vi "Calculate_aomVolts.vi"(8 "error in (no error)":errorcluster, 10 "Power":dbl[](array[numeric])=[0.0, 0.0, 0.0, 0.0] min=0.0 max=1.0, 11 "Fit Parameters":dbl[](array[numeric])=[0.16846, 70.4259, 1.31931]) -> (0 "error out":errorcluster, 2 "AOM Voltage":dbl[](array[numeric]))   [LabVIEW 2016]
uses:
  <vilib>/express/express arith-compare/Formula/XNode/ExpressFormulaBlockNode.xnode
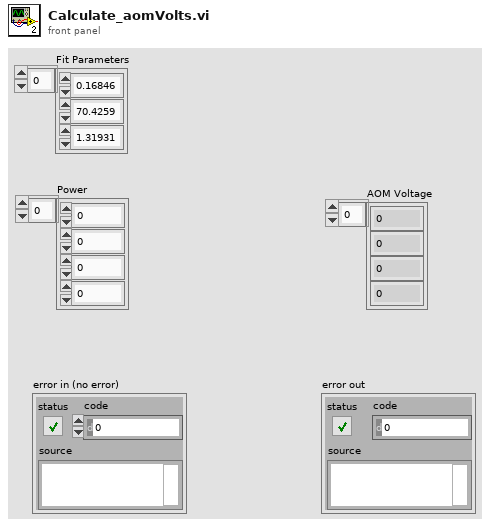
[diagram p1: front panel]
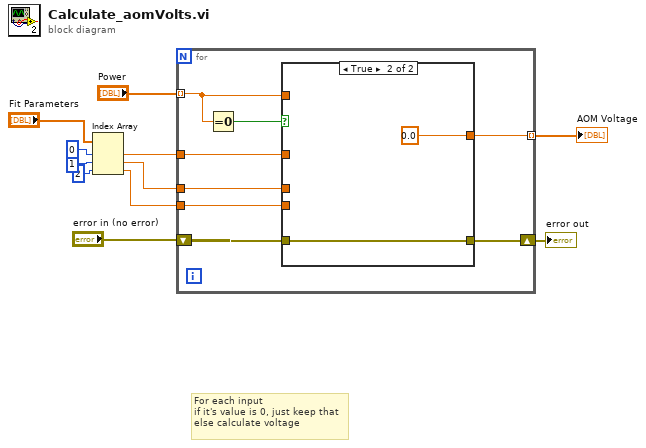
[diagram p0: block diagram]
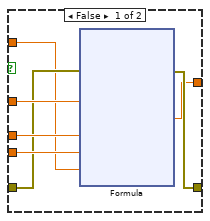
[diagram p2: hidden frame]
diagram:
  # "For each input\nif it's value is 0, just keep that\nelse calculate voltage"
  n1 = Index Array(array="Fit Parameters", index #1=0 ("index"), index #2=1 ("index"), index #3=2 ("index")) -> (element #1=w5:dbl, element #2=w4:dbl, element #3=w3:dbl)
  n2 = for {
    tunnel: w5 -> [w19]
    tunnel: w4 -> [w18]
    tunnel: w3 -> [w17]
    shift-right: [w15] -> w9
    shift-left: "error in (no error)" -> [w16]
    tunnel: "Power" -> [w12] mode=indexing
    tunnel: [w13] -> w1 mode=indexing
    n3 = Equal To 0?(x=w12) -> (x = 0?=w14:bool)
    n4 = case shown="True" w14 {
      tunnel: w19 -> [w26 _]
      tunnel: w18 -> [w25 _]
      tunnel: w17 -> [w24 _]
      tunnel: w16 -> [w23 w41]
      tunnel: [w22 w41] -> w15
      tunnel: [w21 0.0] -> w13
      tunnel: w12 -> [w20 _]
      frame False {
        n5 = xnode "Formula"("X1"=w26, "X2"=w25, "X3"=w24, "P"=w20, "error in (no error)"=w23) -> ("Result"=w21:dbl, "error out"=w22:errorcluster)
      }
      frame True {
      }
    }
  }
  "error out" <- w9
  "AOM Voltage" <- w1
